vi "Periodic Tasks.vi"(8 "error in":errorcluster) -> ()   [LabVIEW 2017]
doc: "This VI runs in parallel to other tasks. It can contain as many user-defined periodic loops as you need. These can carry out PID or other sorts of timed response."
uses:
  <vilib>/Rock Robotics/WPI/Utilities/WPI_GetSetVariantRefNum.vi
  <vilib>/Rock Robotics/WPI/ThirdParty/Phoenix-LabVIEW/Pigeon IMU/CTRE_PigeonIMU_GetYPR.vi
  <vilib>/Rock Robotics/WPI/ThirdParty/Phoenix-LabVIEW/Pigeon IMU/CTRE_PigeonIMU_GetBiasedAccelerometer.vi
  Robot Global Data.vi
  <vilib>/Rock Robotics/Network Tables/NT Write Numeric Array.vi
  <vilib>/Rock Robotics/WPI/ThirdParty/Phoenix-LabVIEW/Motor Controller/Get/CTRE_Phoenix_MotorController_GetSelectedSensorData.vi
  <vilib>/Rock Robotics/WPI/ThirdParty/Phoenix-LabVIEW/Motor Controller/Get/CTRE_Phoenix_MotorController_GetLimitSwitchStates.vi
  <vilib>/Rock Robotics/Network Tables/NT Write Boolean Array.vi
  <vilib>/Rock Robotics/SystemInterfaces/AI/FPGA_AIChannel.ctl
  <vilib>/Rock Robotics/Network Tables/NT Write Number.vi
  <vilib>/Rock Robotics/WPI/Ultrasonic/WPI_SonarMB1010AnalogGetRange.vi
  <vilib>/Rock Robotics/WPI/Ultrasonic/WPI_SonarMB1010AnalogClose.vi
  <vilib>/Rock Robotics/WPI/Ultrasonic/WPI_SonarMB1010AnalogOpen.vi
  <vilib>/Rock Robotics/WPI/Ultrasonic/WPI_SonarMB1010AnalogRefNum Registry Set.vi
panel:
  out "distance":dbl(slide)=125.0 scale=0.0..250.0 scale format="%3d"
  in  "Scaling Factor":dbl=0.025
  in  "Average Bits":u8=3 max=15
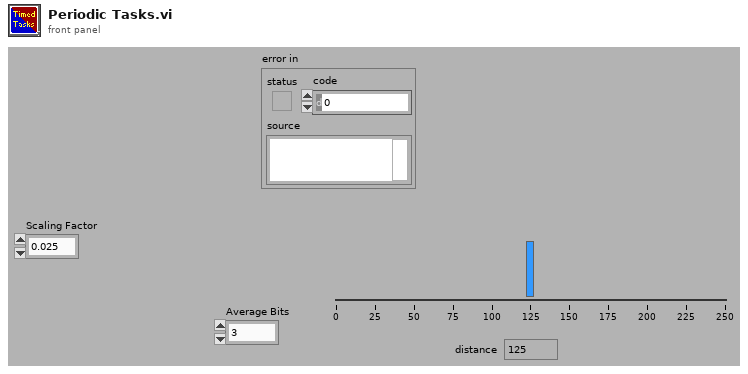
[diagram p1: front panel]
types:
  T1 = typedef "FPGA_AIChannel.ctl" = enum8{"AI 0", "AI 1", "AI 2", "AI 3", "AI MXP 0", "AI MXP 1", "AI MXP 2", "AI MXP 3", "Invalid"}
  T2 = typedef "WPI_SonarMB1010AnalogDeviceRef.ctl" = cluster{"AIDeviceRef":T3, "Scaling factor (V/in)":dbl, "Average Bits":u8}
  T3 = typedef "WPI_AnalogChannelDevRef.ctl" = cluster{"DevStatus":errorcluster, "Analog Channel":T1}
  T4 = typedef "CTRE_PigeonIMU_DeviceRef.ctl" = cluster{"DeviceStatus":errorcluster, "Device Number":u8, "Type":T5, "Device ID":u32, "Handle":u64, "UsageFrame":u32, "Library Path":path}
  T5 = typedef "CTRE_PigeonIMU_ConnectionType.ctl" = u32
  T6 = typedef "WPI_RobotDriveDevRef.ctl" = cluster{"DevStatus":errorcluster, "Motors[]":T7[], "Square Inputs":bool, "Max Output":dbl}
  T7 = typedef "WPI_MotorControlDeviceRef.ctl" = cluster{"DeviceStatus":errorcluster, "Type":T8, "PWM":cluster{"PWM Channel":T9, "DeadBand":T10}, "CAN":cluster{"Device Number":u8, "SetOutput VI Ref":variant, "GetOutput VI Ref":variant, "Enable VI Ref":variant, "Disable VI Ref":variant, "Data":variant}, "Invert":bool, "DIO PWM":cluster{"PWM \"Enable\" Channel":T9, "DIOChannel":T11, "PWM Rate":dbl}}
  T8 = typedef "WPI_MotorControlType.ctl" = enum16{"PWM", "CAN", "DIO PWM"}
  T9 = typedef "FPGA_DIOPWMChannel.ctl" = enum8{"PWM 0", "PWM 1", "PWM 2", "PWM 3", "PWM 4", "PWM 5", "PWM 6", "PWM 7", "PWM 8", "PWM 9", "PWM MXP 0", "PWM MXP 1", "PWM MXP 2", "PWM MXP 3", "PWM MXP 4", "PWM MXP 5", "PWM MXP 6", "PWM MXP 7", "PWM MXP 8", "PWM MXP 9", "Invalid"}
  T10 = typedef "WPI_PWMDeadband.ctl" = cluster{"Name":string, "maxPositivePwm":i32, "minPositivePwm":i32, "centerPwm":i32, "maxNegativePwm":i32, "minNegativePwm":i32, "angularRange":u16}
  T11 = typedef "FPGA_DIOChannel.ctl" = enum8{"DIO 0", "DIO 1", "DIO 2", "DIO 3", "DIO 4", "DIO 5", "DIO 6", "DIO 7", "DIO 8", "DIO 9", "DIO MXP 0", "DIO MXP 1", "DIO MXP 2", "DIO MXP 3", "DIO MXP 4", "DIO MXP 5", "DIO MXP 6", "DIO MXP 7", "DIO MXP 8", "DIO MXP 9", "DIO MXP 10", "DIO MXP 11", "DIO MXP 12", "DIO MXP 13", "DIO MXP 14", "DIO MXP 15", "SPI Port CS1", "SPI Port CS2", "SPI Port CS3", "SPI Port MISO", "SPI Port MOSI", "Invalid"}
  T12 = typedef "WPI_JoystickDevRef.ctl" = cluster{"Device":T13}
  T13 = typedef "WPI_JoystickDeviceEnum.ctl" = enum16{"USB 0", "USB 1", "USB 2", "USB 3", "USB 4", "USB 5"}
  T14 = cluster{"JoystickDevRef":T12, "RobotDriveDevRef":T6}
  T15 = cluster{"Position (Raw Sensor Units)":i32, "Velocity (Raw Sensor Units per 100 ms)":i32}
  T16 = cluster{"Forward Limit Closed?":bool, "Reverse Limit Closed?":bool}
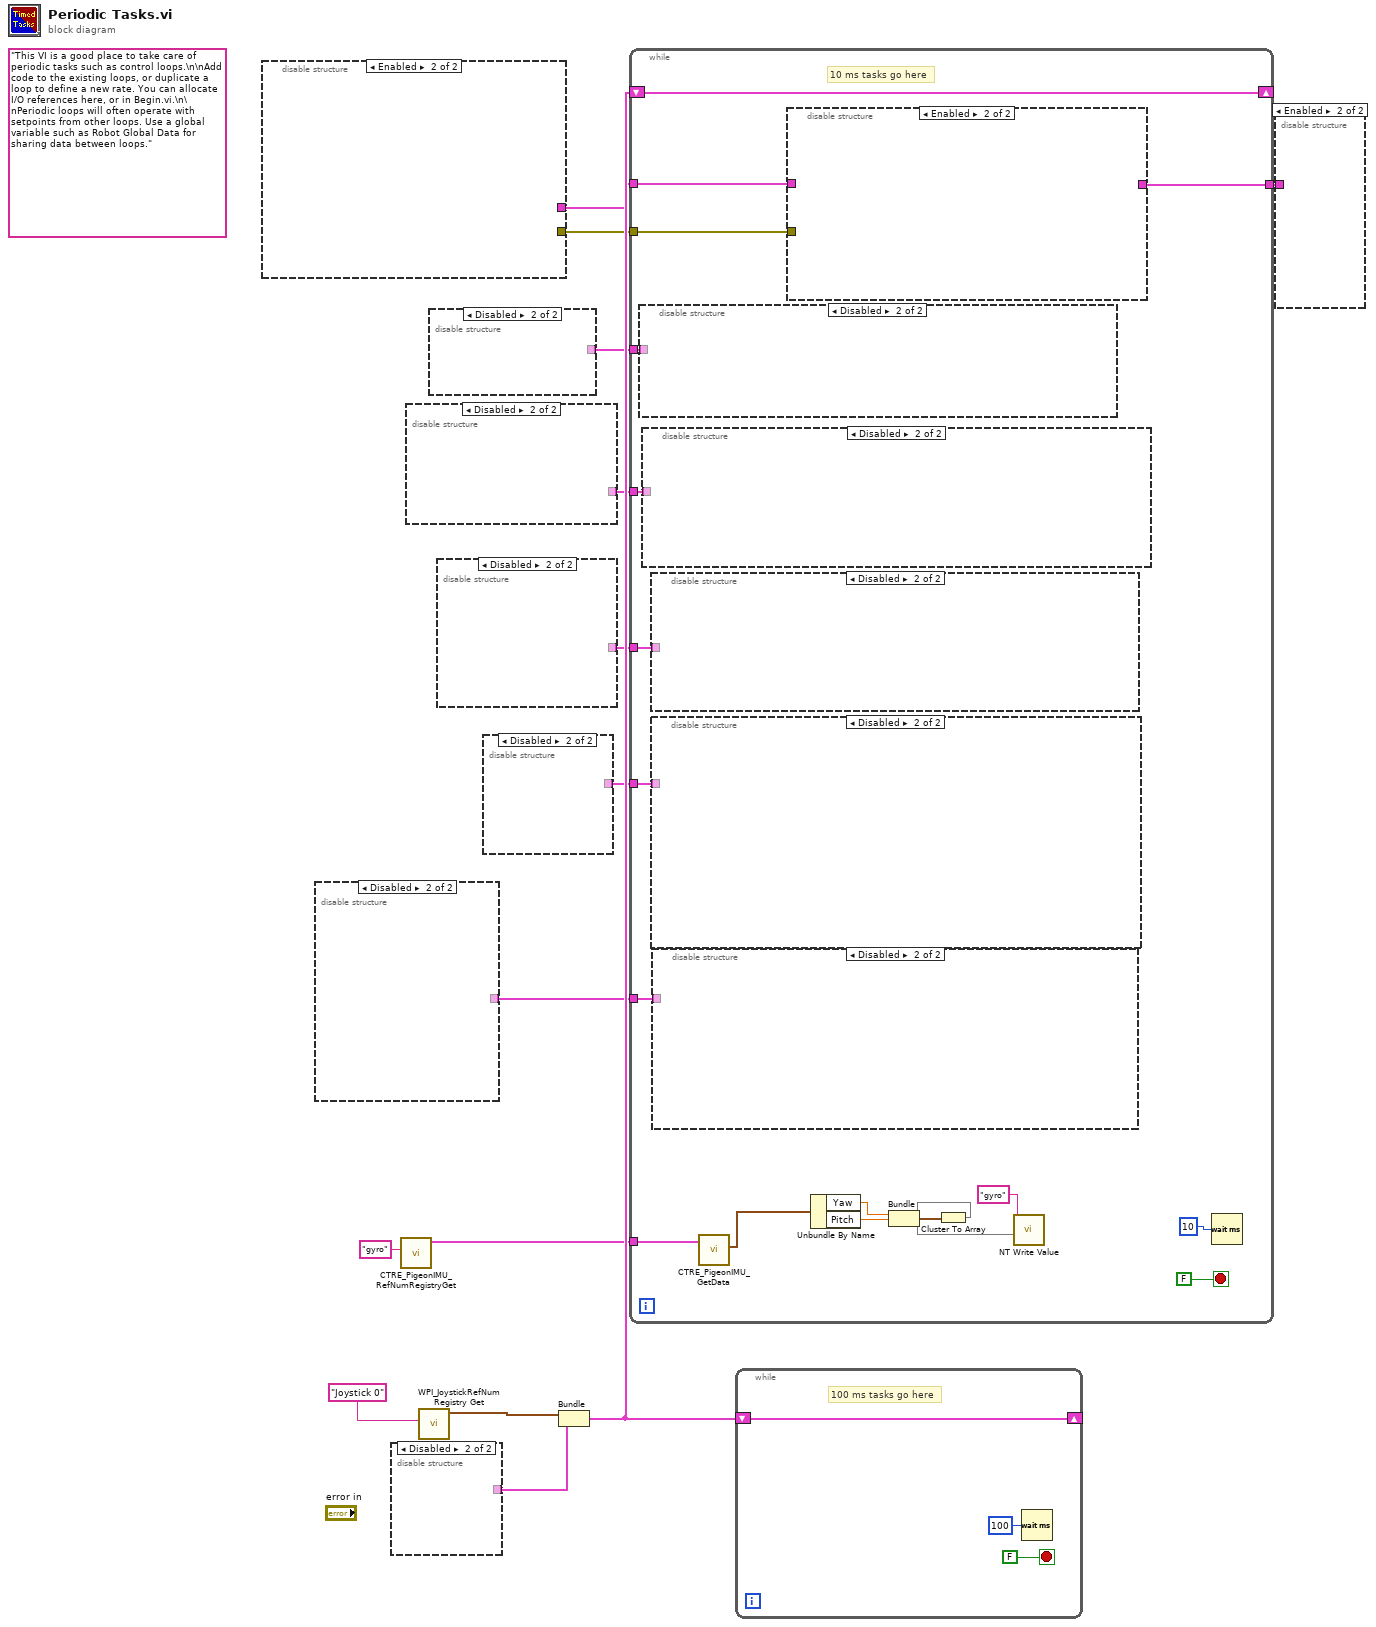
[diagram p0: block diagram]
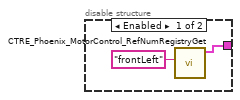
[diagram p2: hidden frame]
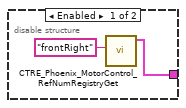
[diagram p3: hidden frame]
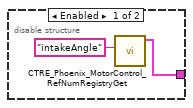
[diagram p4: hidden frame]
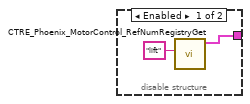
[diagram p5: hidden frame]
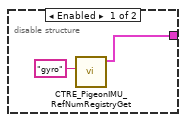
[diagram p6: hidden frame]
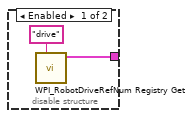
[diagram p7: hidden frame]
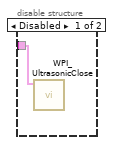
[diagram p8: hidden frame]
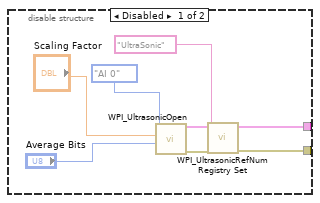
[diagram p9: hidden frame]
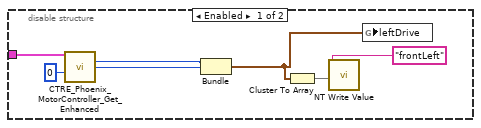
[diagram p10: hidden frame]
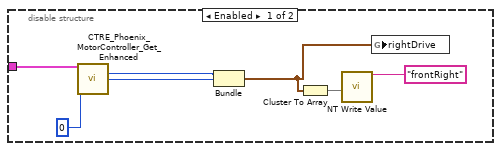
[diagram p11: hidden frame]
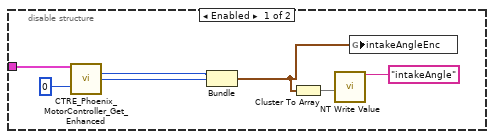
[diagram p12: hidden frame]
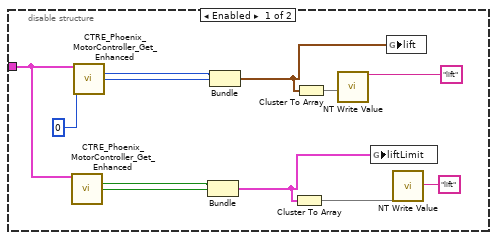
[diagram p13: hidden frame]
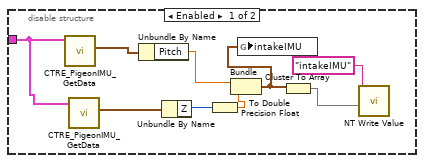
[diagram p14: hidden frame]
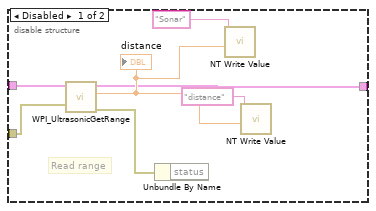
[diagram p15: hidden frame]
diagram:
  (unwired) "This VI is a good place to take care of periodic tasks such as control loops.\n\nAdd code to the existing loops, or duplicate a loop to define a new rate. You can allocate I/O references here, or in Begin.vi.\n\nPeriodic loops will often operate with setpoints from other loops. Use a global variable such as Robot Global Data for sharing data between loops."
  n1 = disable-structure shown="Enabled" {
    disable-tunnel: [w16 _] -> w10
    disable-tunnel: [w15 _] -> w9
    frame Disabled {
      n2 = call-poly <vilib>:"WPI_UltrasonicOpen.vi"("Average Bits"="Average Bits", "Scaling factor (V/in)"="Scaling Factor", "Analog Channel"=FPGA_AIChannel."AI 0") -> ("error out"=w20:errorcluster, "SonarMB1010AnalogDevRef"=w18:T2)  [unwired: 7 in]
      n3 = call-poly <vilib>:"WPI_UltrasonicRefNum Registry Set.vi"("error in (no error)"=w20, "refnum name"="UltraSonic", "SonarMB1010AnalogDevRef"=w18) -> ("error out"=w15:errorcluster, "SonarMB1010AnalogDevRef"=w16:T2)  [unwired: 7 in]
    }
    frame Enabled {
    }
  }
  n4 = disable-structure shown="Disabled" {
    disable-tunnel: [w23 _] -> w1
    frame Enabled {
      n5 = call <vilib>:"CTRE_PigeonIMU_RefNumRegistryGet.vi"("refnum name"="gyro") -> ("PigeonIMUDevRef"=w23:T4)  [unwired: 9 in, 1 out]
    }
    frame Disabled {
    }
  }
  n6 = disable-structure shown="Disabled" {
    disable-tunnel: [w25 _] -> w12
    frame Enabled {
      n7 = call <vilib>:"WPI_RobotDriveRefNum Registry Get.vi"("refnum name"="drive") -> ("RobotDriveDevRef"=w25:T6)  [unwired: 1 in, 9 out]
    }
    frame Disabled {
    }
  }
  n8 = call <vilib>:"CTRE_PigeonIMU_RefNumRegistryGet.vi"("refnum name"="gyro") -> ("PigeonIMUDevRef"=w2:T4)  [unwired: 9 in, 1 out]
  n9 = disable-structure shown="Disabled" {
    disable-tunnel: [w27 _] -> w5
    frame Enabled {
      n10 = call <vilib>:"CTRE_Phoenix_MotorControl_RefNumRegistryGet.vi"("refnum name"="frontRight") -> ("PhoenixMotorControlDevRef"=w27:T7)  [unwired: 9 in, 1 out]
    }
    frame Disabled {
    }
  }
  n11 = call <vilib>:"WPI_JoystickRefNum Registry Get.vi"("refnum name"="Joystick 0") -> ("JoystickDevRef"=w13:T12)  [unwired: 1 in, 9 out]
  n12 = disable-structure shown="Disabled" {
    disable-tunnel: [w29 _] -> w6
    frame Enabled {
      n13 = call <vilib>:"CTRE_Phoenix_MotorControl_RefNumRegistryGet.vi"("refnum name"="frontLeft") -> ("PhoenixMotorControlDevRef"=w29:T7)  [unwired: 9 in, 1 out]
    }
    frame Disabled {
    }
  }
  n14 = disable-structure shown="Disabled" {
    disable-tunnel: [w32 _] -> w4
    frame Enabled {
      n15 = call <vilib>:"CTRE_Phoenix_MotorControl_RefNumRegistryGet.vi"("refnum name"="intakeAngle") -> ("PhoenixMotorControlDevRef"=w32:T7)  [unwired: 9 in, 1 out]
    }
    frame Disabled {
    }
  }
  n16 = disable-structure shown="Disabled" {
    disable-tunnel: [w33 _] -> w3
    frame Enabled {
      n17 = call <vilib>:"CTRE_Phoenix_MotorControl_RefNumRegistryGet.vi"("refnum name"="lift") -> ("PhoenixMotorControlDevRef"=w33:T7)  [unwired: 9 in, 1 out]
    }
    frame Disabled {
    }
  }
  n18 = Bundle("JoystickDevRef"=w13, "RobotDriveDevRef"=w12) -> (w11:T14)  [unwired: 1 out]
  n19 = while {
    shift-right: [w50] -> _
    shift-left: w11 -> [w50]
    tunnel: w10 -> [w49]
    tunnel: w9 -> [w48]
    tunnel: [w47] -> w8
    tunnel: w6 -> [w45]
    tunnel: w5 -> [w44]
    tunnel: w4 -> [w43]
    tunnel: w3 -> [w42]
    tunnel: w2 -> [w37]
    tunnel: w1 -> [w35]
    stop <- FALSE stop-if-true
    # "10 ms tasks go here"
    n20 = disable-structure shown="Disabled" {
      disable-tunnel: w45 -> [w59 _]
      frame Enabled {
        n21 = call-poly <vilib>:"CTRE_Phoenix_MotorController_Get_Enhanced.vi"("PhoenixMotorControlDevRef"=w59, "pidLoopIdx"=u32 0) -> ("Position (Raw Sensor Units)"=w57:i32, "Velocity (Raw Sensor Units per 100 ms)"=w56:i32)  [unwired: 10 in, 2 out]
        n22 = Bundle("Position (Raw Sensor Units)"=w57, "Velocity (Raw Sensor Units per 100 ms)"=w56) -> (w53:T15)  [unwired: 1 in]
        n23 = Cluster To Array(cluster=w53) -> (array=w55:i32[])
        n24 = call-poly <vilib>:"NT Write Value.vi"("Numeric Array"=w55, "Name"="frontLeft") -> ()  [unwired: 9 in, 1 out]
        n25 = global write "Robot Global Data.vi" "leftDrive"(w53) -> ()
      }
      frame Disabled {
      }
    }
    n26 = disable-structure shown="Disabled" {
      disable-tunnel: w44 -> [w60 _]
      frame Enabled {
        n27 = call-poly <vilib>:"CTRE_Phoenix_MotorController_Get_Enhanced.vi"("PhoenixMotorControlDevRef"=w60, "pidLoopIdx"=u32 0) -> ("Position (Raw Sensor Units)"=w62:i32, "Velocity (Raw Sensor Units per 100 ms)"=w63:i32)  [unwired: 10 in, 2 out]
        n28 = Bundle("Position (Raw Sensor Units)"=w62, "Velocity (Raw Sensor Units per 100 ms)"=w63) -> (w66:T15)  [unwired: 1 in]
        n29 = Cluster To Array(cluster=w66) -> (array=w64:i32[])
        n30 = call-poly <vilib>:"NT Write Value.vi"("Numeric Array"=w64, "Name"="frontRight") -> ()  [unwired: 9 in, 1 out]
        n31 = global write "Robot Global Data.vi" "rightDrive"(w66) -> ()
      }
      frame Disabled {
      }
    }
    n32 = disable-structure shown="Disabled" {
      disable-tunnel: w43 -> [w73 _]
      frame Enabled {
        n33 = call-poly <vilib>:"CTRE_Phoenix_MotorController_Get_Enhanced.vi"("PhoenixMotorControlDevRef"=w73, "pidLoopIdx"=u32 0) -> ("Position (Raw Sensor Units)"=w71:i32, "Velocity (Raw Sensor Units per 100 ms)"=w70:i32)  [unwired: 10 in, 2 out]
        n34 = Bundle("Position (Raw Sensor Units)"=w71, "Velocity (Raw Sensor Units per 100 ms)"=w70) -> (w67:T15)  [unwired: 1 in]
        n35 = Cluster To Array(cluster=w67) -> (array=w69:i32[])
        n36 = call-poly <vilib>:"NT Write Value.vi"("Numeric Array"=w69, "Name"="intakeAngle") -> ()  [unwired: 9 in, 1 out]
        n37 = global write "Robot Global Data.vi" "intakeAngleEnc"(w67) -> ()
      }
      frame Disabled {
      }
    }
    n38 = disable-structure shown="Disabled" {
      disable-tunnel: w42 -> [w74 _]
      frame Enabled {
        n39 = call-poly <vilib>:"CTRE_Phoenix_MotorController_Get_Enhanced.vi"("PhoenixMotorControlDevRef"=w74) -> ("Forward Limit Closed?"=w79:bool, "Reverse Limit Closed?"=w78:bool)  [unwired: 11 in, 2 out]
        n40 = call-poly <vilib>:"CTRE_Phoenix_MotorController_Get_Enhanced.vi"("PhoenixMotorControlDevRef"=w74, "pidLoopIdx"=u32 0) -> ("Position (Raw Sensor Units)"=w81:i32, "Velocity (Raw Sensor Units per 100 ms)"=w82:i32)  [unwired: 10 in, 2 out]
        n41 = Bundle("Forward Limit Closed?"=w79, "Reverse Limit Closed?"=w78) -> (w75:T16)  [unwired: 1 in]
        n42 = Bundle("Position (Raw Sensor Units)"=w81, "Velocity (Raw Sensor Units per 100 ms)"=w82) -> (w85:T15)  [unwired: 1 in]
        n43 = Cluster To Array(cluster=w75) -> (array=w77:bool[])
        n44 = Cluster To Array(cluster=w85) -> (array=w83:i32[])
        n45 = call-poly <vilib>:"NT Write Value.vi"("Numeric Array"=w83, "Name"="lift") -> ()  [unwired: 9 in, 1 out]
        n46 = global write "Robot Global Data.vi" "liftLimit"(w75) -> ()
        n47 = global write "Robot Global Data.vi" "lift"(w85) -> ()
        n48 = call-poly <vilib>:"NT Write Value.vi"("Boolean Array"=w77, "Name"="lift") -> ()  [unwired: 9 in, 1 out]
      }
      frame Disabled {
      }
    }
    n49 = disable-structure shown="Disabled" {
      disable-tunnel: w35 -> [w89 _]
      frame Enabled {
        n50 = call-poly <vilib>:"CTRE_PigeonIMU_GetData.vi"("PigeonIMUDevRef"=w89) -> ("Yaw Pitch Roll"=w93:cluster{"Yaw":dbl, "Pitch":dbl, "Roll":dbl})  [unwired: 8 in, 2 out]
        n51 = call-poly <vilib>:"CTRE_PigeonIMU_GetData.vi"("PigeonIMUDevRef"=w89) -> ("Biased Accelerometer"=w90:cluster{"X":i16, "Y":i16, "Z":i16, "Norm":i16})  [unwired: 8 in, 2 out]
        n52 = Unbundle By Name(w93) -> ("Pitch"=w92:dbl)
        n53 = Unbundle By Name(w90) -> ("Z"=w88:i16)
        n54 = To Double Precision Float(number=w88) -> (double precision float=w87:dbl)
        n55 = Bundle("Pitch"=w92, w87) -> (w86:cluster{"Pitch":dbl, dbl})  [unwired: 1 in]
        n56 = global write "Robot Global Data.vi" "intakeIMU"(w86) -> ()
        n57 = Cluster To Array(cluster=w86) -> (array=w91:dbl[])
        n58 = call-poly <vilib>:"NT Write Value.vi"("Numeric Array"=w91, "Name"="intakeIMU") -> ()  [unwired: 9 in, 1 out]
      }
      frame Disabled {
      }
    }
    n59 = call-poly <vilib>:"CTRE_PigeonIMU_GetData.vi"("PigeonIMUDevRef"=w37) -> ("Yaw Pitch Roll"=w36:cluster{"Yaw":dbl, "Pitch":dbl, "Roll":dbl})  [unwired: 8 in, 2 out]
    n60 = disable-structure shown="Enabled" {
      disable-tunnel: w49 -> [w97 _]
      disable-tunnel: w48 -> [w96 _]
      disable-tunnel: [w95 _] -> w47
      frame Disabled {
        # "Read range"
        n61 = call-poly <vilib>:"WPI_UltrasonicGetRange.vi"("error in"=w96, "SonarMB1010AnalogDevRef"=w97) -> ("error out"=w101:errorcluster, "Distance"=w99:dbl, "SonarMB1010AnalogDevRef"=w95:T2)  [unwired: 7 in]
        "distance" <- w99
        n62 = Unbundle By Name(w101) -> ()  [unwired: 1 out]
        n63 = call-poly <vilib>:"NT Write Value.vi"("Numeric"=w99, "Name"="Sonar") -> ()  [unwired: 9 in, 1 out]
        n64 = call-poly <vilib>:"NT Write Value.vi"("Numeric"=w99, "Name"="distance") -> ()  [unwired: 9 in, 1 out]
      }
      frame Enabled {
      }
    }
    n65 = Unbundle By Name(w36) -> ("Yaw"=w40:dbl, "Pitch"=w41:dbl)
    n66 = Bundle("Yaw"=w40, "Pitch"=w41) -> (w39:cluster{"Yaw":dbl, "Pitch":dbl})  [unwired: 1 in]
    n67 = Cluster To Array(cluster=w39) -> (array=w38:dbl[])
    n68 = call-poly <vilib>:"NT Write Value.vi"("Numeric Array"=w38, "Name"="gyro") -> ()  [unwired: 9 in, 1 out]
    n69 = Wait (ms)(milliseconds to wait=u32 10) -> ()  [unwired: 1 out]
  }
  n70 = while {
    shift-right: [w102] -> _
    shift-left: w11 -> [w102]
    stop <- FALSE stop-if-true
    # "100 ms tasks go here"
    n71 = Wait (ms)(milliseconds to wait=u32 100) -> ()  [unwired: 1 out]
  }
  n72 = disable-structure shown="Enabled" {
    disable-tunnel: w8 -> [w105 _]
    frame Disabled {
      n73 = call-poly <vilib>:"WPI_UltrasonicClose.vi"("SonarMB1010AnalogDevRef"=w105) -> ()  [unwired: 10 in, 1 out]
    }
    frame Enabled {
    }
  }
